vi "refresh comparison UI.vi"(6 "engine configuration":refnum<class "engine configuration.lvclass">, 7 "comparisons":T1[](array[typedef]), 8 "error in\\":errorcluster, 9 "output":refnum<class "TBM channel.lvclass">, 10 "unlatch":refnum<class "TBM channel.lvclass">, 11 "tag select module configuration in":refnum<class "tag select module configuration.lvclass">) -> (0 "error out":errorcluster, 1 "unlatch tag":string, 2 "Item Names":string[](array[string]), 5 "output tag":string)   [LabVIEW 2013]
uses:
  <vilib>/NI/Module Execution Interface/Engine Configuration/engine configuration.lvclass
  module/configuration/alarm comparison.ctl
  <vilib>/NI/Tag Bus Module Framework/channel/TBM channel.lvclass
  module/configuration/compare type.ctl
  module/configuration/tag select module configuration.lvclass
  <vilib>/NI/Configuration Framework/serializable configuration/NISE_CEF_serializable configuration.lvclass/NISE_CEF_serializable configuration.ctl
  <vilib>/NI/Tag Bus/tag/tag descriptor.lvclass/tag descriptor.ctl
  <vilib>/NI/Tag Bus/tag/read tag name.vi
  <vilib>/NI/Configuration Framework/serializable configuration/Read UID.vi
  <vilib>/Utility/LVClass/Get LV Class Name.vi
  <vilib>/NI/Configuration Framework/error generator/NISE_error generator.vi
  <vilib>/NI/Tag Bus/tag/tag descriptor.lvclass
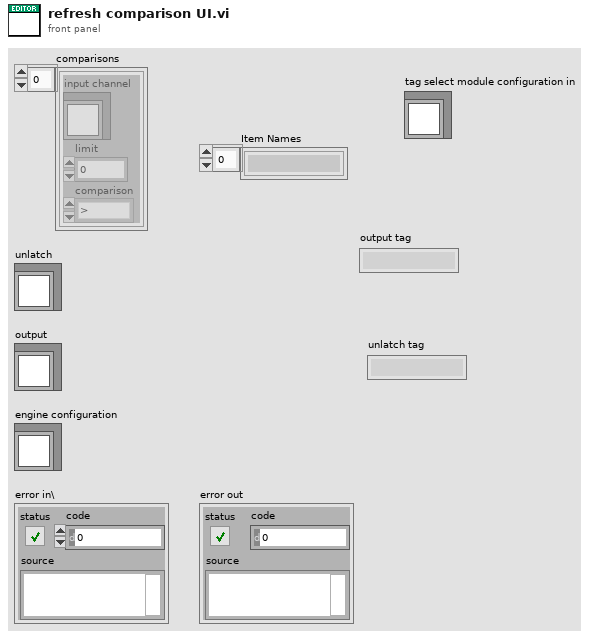
[diagram p1: front panel]
types:
  T1 = typedef "alarm comparison.ctl" = cluster{"input channel":refnum<class "TBM channel.lvclass">, "limit":dbl, "comparison":T2}
  T2 = typedef "compare type.ctl" = enum16{">", "<", ">=", "<=", "="}
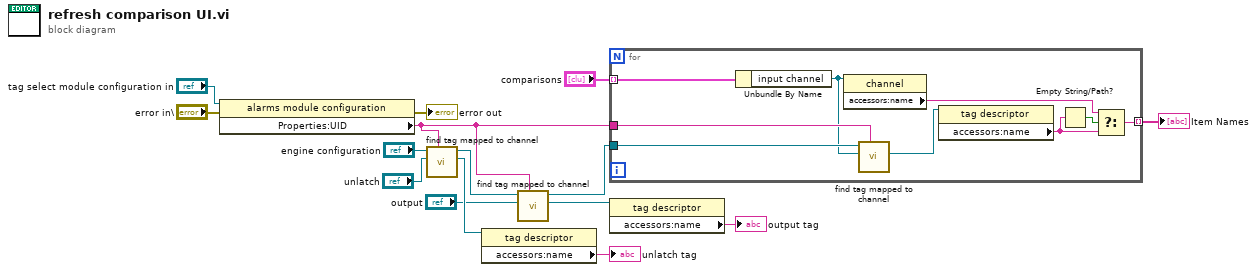
[diagram p0: block diagram]
diagram:
  n1 = property class="alarms module configuration"(reference="tag select module configuration in", error in="error in\\") -> (error out=→"error out":errorcluster, "Properties:UID"=w2:string)  [unwired: 1 out]
  n2 = call <vilib>:"find tag mapped to channel.vi"("owner"=w2, "channel"="unlatch", "engine configuration in"="engine configuration") -> ("tag"=w9:refnum<class "tag descriptor.lvclass">, "engine configuration out"=w12:refnum<class "engine configuration.lvclass">)  [unwired: 6 in, 1 out]
  n3 = property class="tag descriptor"(reference=w9) -> ("accessors:name"=→"unlatch tag":string)  [unwired: 1 in, 2 out]
  n4 = call <vilib>:"find tag mapped to channel.vi"("owner"=w2, "channel"="output", "engine configuration in"=w12) -> ("tag"=w7:refnum<class "tag descriptor.lvclass">, "engine configuration out"=w3:refnum<class "engine configuration.lvclass">)  [unwired: 6 in, 1 out]
  n5 = for {
    tunnel: "comparisons" -> [w24] mode=indexing
    tunnel: w3 -> [w23]
    tunnel: w2 -> [w22]
    tunnel: [w18] -> w1 mode=indexing
    n6 = Unbundle By Name(w24) -> ("input channel"=w17:refnum<class "TBM channel.lvclass">)
    n7 = property class="channel"(reference=w17) -> ("accessors:name"=w16:string)  [unwired: 1 in, 2 out]
    n8 = call <vilib>:"find tag mapped to channel.vi"("owner"=w22, "channel"=w17, "engine configuration in"=w23) -> ("tag"=w21:refnum<class "tag descriptor.lvclass">)  [unwired: 6 in, 2 out]
    n9 = property class="tag descriptor"(reference=w21) -> ("accessors:name"=w19:string)  [unwired: 1 in, 2 out]
    n10 = Empty String/Path?(string/path=w19) -> (empty?=w20:bool)
    n11 = Select(t=w16, s=w20, f=w19) -> (s? t:f=w18:string)
  }
  "Item Names" <- w1
  n12 = property class="tag descriptor"(reference=w7) -> ("accessors:name"=→"output tag":string)  [unwired: 1 in, 2 out]
